vi "AC_2F1_ctl.vi"(8 "error in":errorcluster caption="错误输入（无错误）", 9 "Input2":T2, 11 "Input1":T3) -> (0 "error out":errorcluster caption="错误输出", 1 "AC2F1":T1 {"驻车空调失效状态" items=["失效", "未失效", "预留"]; "驻车空调状态" items=["关闭", "开启", "预留", "无效"]; "PM2.5传感器工作状态" items=["初始态", "数据收集中", "完成", "关闭"]; "室内空气质量等级" items=["Level1", "Level2", "Level3", "Level4", "Level5", "Level6", "预留", "无效"]; "室外空气PM2.5浓度" min=0 max=999 step=1 scale=0.0..999.0; "室内空气PM2.5浓度" min=0 max=999 step=1 scale=0.0..999.0; "AC大气温度传感器读数" min=-40.0 max=60.0 step=0.5 scale=-40.0..60.0}, 3 "CmdStr":string)   [LabVIEW 2013]
uses:
  Input1.ctl
  Input2.ctl
  AC_2F1.ctl
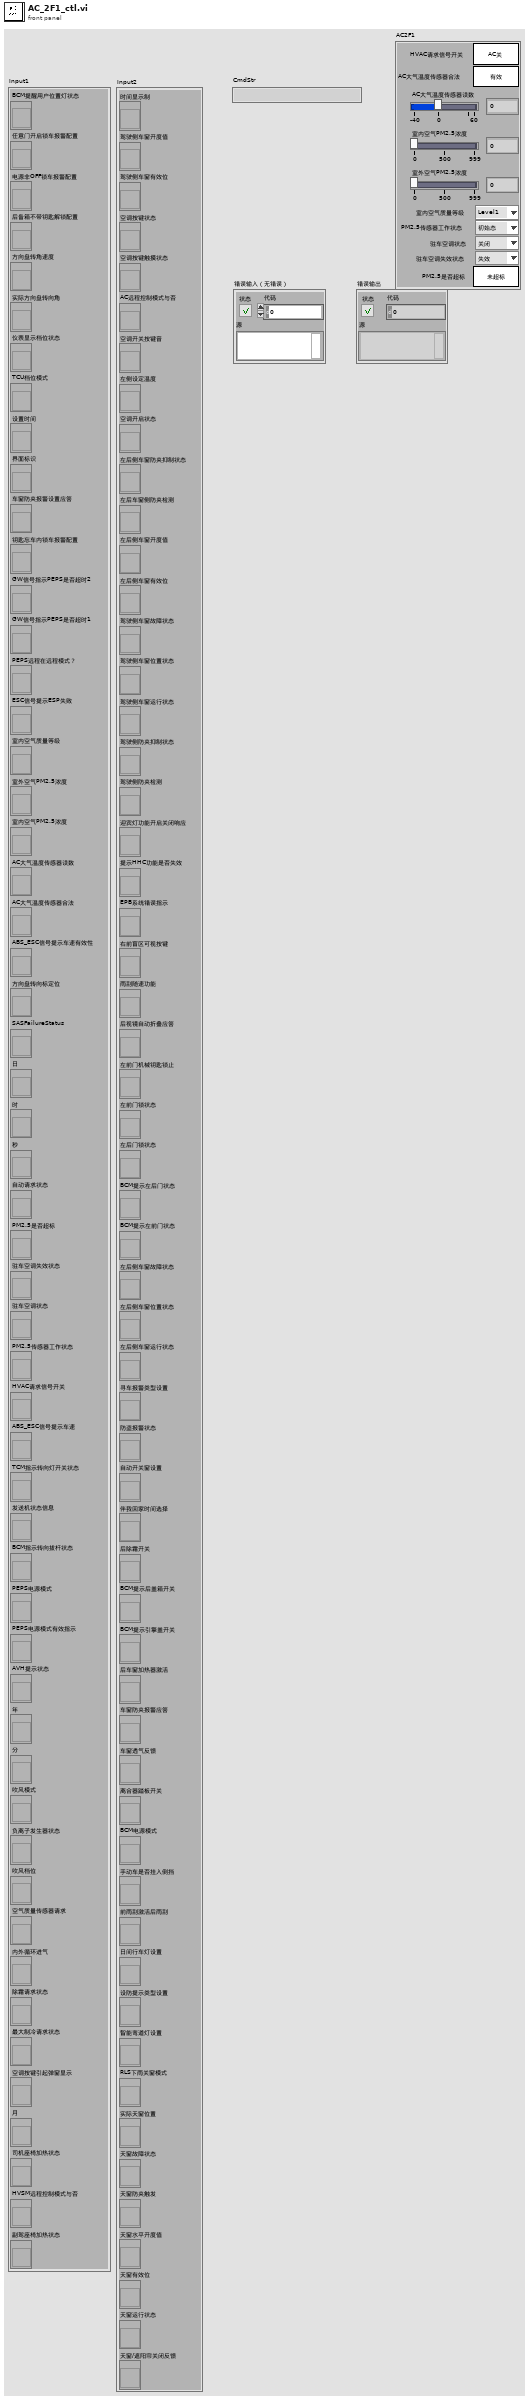
[diagram p1: front panel]
types:
  T1 = typedef "AC_2F1.ctl" = cluster{"HVAC请求信号开关":bool, "AC大气温度传感器合法":bool, "AC大气温度传感器读数":dbl, "室内空气PM2.5浓度":i32, "室外空气PM2.5浓度":i32, "室内空气质量等级":u16, "PM2.5传感器工作状态":u16, "驻车空调状态":u16, "驻车空调失效状态":u16, "PM2.5是否超标":bool}
  T2 = typedef "Input2.ctl" = cluster{"时间显示制":refnum<vi>, "驾驶侧车窗开度值":refnum<vi>, "驾驶侧车窗有效位":refnum<vi>, "空调按键状态":refnum<vi>, "空调按键触摸状态":refnum<vi>, "AC远程控制模式与否":refnum<vi>, "空调开关按键音":refnum<vi>, "左侧设定温度":refnum<vi>, "空调开启状态":refnum<vi>, "左后侧车窗防夹抑制状态":refnum<vi>, "左后车窗侧防夹检测":refnum<vi>, "左后侧车窗开度值":refnum<vi>, "左后侧车窗有效位":refnum<vi>, "驾驶侧车窗故障状态":refnum<vi>, "驾驶侧车窗位置状态":refnum<vi>, "驾驶侧车窗运行状态":refnum<vi>, "驾驶侧防夹抑制状态":refnum<vi>, "驾驶侧防夹检测":refnum<vi>, "迎宾灯功能开启关闭响应":refnum<vi>, "提示HHC功能是否失效":refnum<vi>, "EPB系统错误指示":refnum<vi>, "右前盲区可视按键":refnum<vi>, "雨刮随速功能":refnum<vi>, "后视镜自动折叠应答":refnum<vi>, "左前门机械钥匙锁止":refnum<vi>, "左前门锁状态":refnum<vi>, "左后门锁状态":refnum<vi>, "BCM提示左后门状态":refnum<vi>, "BCM提示左前门状态":refnum<vi>, "左后侧车窗故障状态":refnum<vi>, "左后侧车窗位置状态":refnum<vi>, "左后侧车窗运行状态":refnum<vi>, "寻车报警类型设置":refnum<vi>, "防盗报警状态":refnum<vi>, "自动开关窗设置":refnum<vi>, "伴我回家时间选择":refnum<vi>, "后除霜开关":refnum<vi>, "BCM提示后盖箱开关":refnum<vi>, "BCM提示引擎盖开关":refnum<vi>, "后车窗加热器激活":refnum<vi>, "车窗防夹报警应答":refnum<vi>, "车窗透气反馈":refnum<vi>, "离合器踏板开关":refnum<vi>, "BCM电源模式":refnum<vi>, "手动车是否挂入倒挡":refnum<vi>, "前雨刮激活后雨刮":refnum<vi>, "日间行车灯设置":refnum<vi>, "设防提示类型设置":refnum<vi>, "智能弯道灯设置":refnum<vi>, "RLS下雨关窗模式":refnum<vi>, "实际天窗位置":refnum<vi>, "天窗故障状态":refnum<vi>, "天窗防夹触发":refnum<vi>, "天窗水平开度值":refnum<vi>, "天窗有效位":refnum<vi>, "天窗运行状态":refnum<vi>, "天窗/遮阳帘关闭反馈":refnum<vi>}
  T3 = typedef "Input1.ctl" = cluster{"BCM提醒用户位置灯状态":refnum<vi>, "任意门开启锁车报警配置":refnum<vi>, "电源非OFF锁车报警配置":refnum<vi>, "后备箱不带钥匙解锁配置":refnum<vi>, "方向盘转角速度":refnum<vi>, "实际方向盘转向角":refnum<vi>, "仪表显示档位状态":refnum<vi>, "TCU档位模式":refnum<vi>, "设置时间":refnum<vi>, "界面标识":refnum<vi>, "车窗防夹报警设置应答":refnum<vi>, "钥匙忘车内锁车报警配置":refnum<vi>, "GW信号指示PEPS是否超时2":refnum<vi>, "GW信号指示PEPS是否超时1":refnum<vi>, "PEPS远程在远程模式？":refnum<vi>, "ESC信号提示ESP失败":refnum<vi>, "室内空气质量等级":refnum<vi>, "室外空气PM2.5浓度":refnum<vi>, "室内空气PM2.5浓度":refnum<vi>, "AC大气温度传感器读数":refnum<vi>, "AC大气温度传感器合法":refnum<vi>, "ABS_ESC信号提示车速有效性":refnum<vi>, "方向盘转向标定位":refnum<vi>, "SASFailureStatus":refnum<vi>, "日":refnum<vi>, "时":refnum<vi>, "秒":refnum<vi>, "自动请求状态":refnum<vi>, "PM2.5是否超标":refnum<vi>, "驻车空调失效状态":refnum<vi>, "驻车空调状态":refnum<vi>, "PM2.5传感器工作状态":refnum<vi>, "HVAC请求信号开关":refnum<vi>, "ABS_ESC信号提示车速":refnum<vi>, "TCM指示转向灯开关状态":refnum<vi>, "发送机状态信息":refnum<vi>, "BCM指示转向拔杆状态":refnum<vi>, "PEPS电源模式":refnum<vi>, "PEPS电源模式有效指示":refnum<vi>, "AVH提示状态":refnum<vi>, "年":refnum<vi>, "分":refnum<vi>, "吹风模式":refnum<vi>, "负离子发生器状态":refnum<vi>, "吹风档位":refnum<vi>, "空气质量传感器请求":refnum<vi>, "内外循环进气":refnum<vi>, "除霜请求状态":refnum<vi>, "最大制冷请求状态":refnum<vi>, "空调按键引起弹窗显示":refnum<vi>, "月":refnum<vi>, "司机座椅加热状态":refnum<vi>, "HVSM远程控制模式与否":refnum<vi>, "副驾座椅加热状态":refnum<vi>}
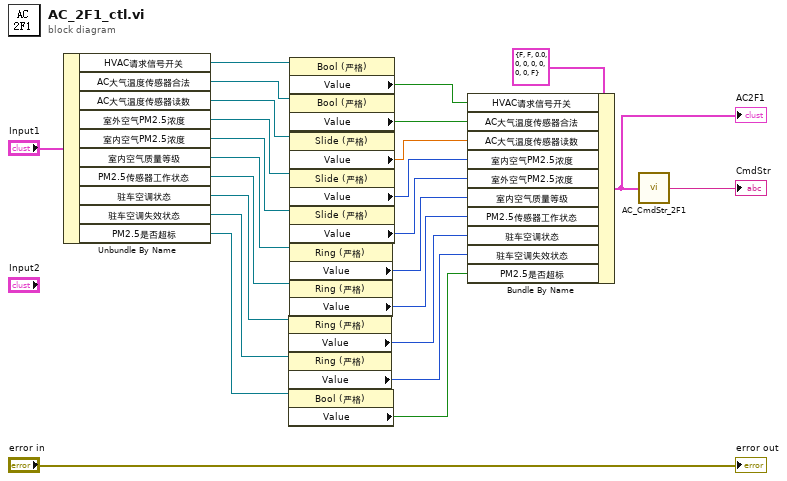
[diagram p0: block diagram]
diagram:
  n1 = Unbundle By Name("Input1") -> ("HVAC请求信号开关"=w22:refnum<vi>, "AC大气温度传感器合法"=w20:refnum<vi>, "AC大气温度传感器读数"=w18:refnum<vi>, "室外空气PM2.5浓度"=w16:refnum<vi>, "室内空气PM2.5浓度"=w14:refnum<vi>, "室内空气质量等级"=w12:refnum<vi>, "PM2.5传感器工作状态"=w10:refnum<vi>, "驻车空调状态"=w8:refnum<vi>, "驻车空调失效状态"=w7:refnum<vi>, "PM2.5是否超标"=w4:refnum<vi>)
  n2 = property class="Ring (严格)"(reference=w8) -> ("Value"=w6:u16)  [unwired: 1 in, 2 out]
  n3 = property class="Ring (严格)"(reference=w7) -> ("Value"=w5:u16)  [unwired: 1 in, 2 out]
  n4 = property class="Bool (严格)"(reference=w4) -> ("Value"=w3:bool)  [unwired: 1 in, 2 out]
  n5 = property class="Bool (严格)"(reference=w22) -> ("Value"=w21:bool)  [unwired: 1 in, 2 out]
  n6 = property class="Bool (严格)"(reference=w20) -> ("Value"=w19:bool)  [unwired: 1 in, 2 out]
  n7 = property class="Slide (严格)"(reference=w18) -> ("Value"=w17:dbl)  [unwired: 1 in, 2 out]
  n8 = property class="Slide (严格)"(reference=w16) -> ("Value"=w15:i32)  [unwired: 1 in, 2 out]
  n9 = property class="Slide (严格)"(reference=w14) -> ("Value"=w13:i32)  [unwired: 1 in, 2 out]
  n10 = property class="Ring (严格)"(reference=w12) -> ("Value"=w11:u16)  [unwired: 1 in, 2 out]
  n11 = property class="Ring (严格)"(reference=w10) -> ("Value"=w9:u16)  [unwired: 1 in, 2 out]
  n12 = Bundle By Name(cluster=T1 {"HVAC请求信号开关"=FALSE, "AC大气温度传感器合法"=FALSE, "AC大气温度传感器读数"=0.0, "室内空气PM2.5浓度"=0, "室外空气PM2.5浓度"=0, "室内空气质量等级"=0, "PM2.5传感器工作状态"=0, "驻车空调状态"=0, "驻车空调失效状态"=0, "PM2.5是否超标"=FALSE} ("AC命令输入"), "HVAC请求信号开关"=w21, "AC大气温度传感器合法"=w19, "AC大气温度传感器读数"=w17, "室内空气PM2.5浓度"=w15, "室外空气PM2.5浓度"=w13, "室内空气质量等级"=w11, "PM2.5传感器工作状态"=w9, "驻车空调状态"=w6, "驻车空调失效状态"=w5, "PM2.5是否超标"=w3) -> (w24:T1)
  "AC2F1" <- w24
  n13 = call "AC_CmdStr_2F1.vi"("AC命令输入"=w24) -> ("CmdStr"=→"CmdStr":string)
  "error out" <- "error in"
